vi "svx_Waterfall Facade.vi"(0 "Data In":T3={"z0"=0.0, "dz"=1.0, "Plots"=[]}, 2 "Display State In":T6={"X Scale Width %"=50.0, "Y Scale Height %"=50.0, "X-Axis Range"={"Minimum"=0.0, "Maximum"=10.0}, "Y-Axis Range"={"Minimum"=0.0, "Maximum"=10.0}, "Z-Axis Range"={"Minimum"=0.0, "Maximum"=10.0}, "Plot Color"=61212, "Frame Color"=16252785, "Background Color"=16777222, "Initial AutoScale Y"=TRUE, "AutoScale X"=2, "AutoScale Y"=2, "AutoScale Z"=2, "Plot Transparency"=FALSE, "X-Axis Name"="Frequency", "Y-Axis Name"="Amplitude", "Z-Axis Name"="", "X-Axis Scaling Factor"={"Offset"=0.0, "Multiplier"=1.0}, "Y-Axis Scaling Factor"={"Offset"=0.0, "Multiplier"=1.0}, "Z-Axis Scaling Factor"={"Offset"=0.0, "Multiplier"=1.0}, "X-Scale Visible"=TRUE, "Y-Scale Visible"=TRUE, "Z-Scale Visible"=TRUE, "X-Scale Label Visible"=TRUE, "Y-Scale Label Visible"=TRUE, "Z-Scale Label Visible"=TRUE, "X-Axis Range Scaled"={"Minimum"=0.0, "Maximum"=10.0}, "Y-Axis Range Scaled"={"Minimum"=0.0, "Maximum"=10.0}, "Z-Axis Range Scaled"={"Minimum"=0.0, "Maximum"=10.0}, "Rev Z Order"=FALSE, "X-Scale Format Str"="%#.4g", "Y-Scale Format Str"="%#.4g", "Z-Scale Format Str"="%#.4g", "Decor color"=12369084, "Scale Range Change"=refnum, "out of state queue"=refnum, "property nodes"=refnum, "Lines"=[], "Line Properties"={"Line Color"=61212, "Line Width"=61212, "Line Style"=enum."Dash", "DisplayLines"=FALSE}} {"Line Properties"."Line Width" min=1}, 3 "Container State":T7) -> (6 "Data Out":T3={"z0"=0.0, "dz"=1.0, "Plots"=[]}, 7 "Display State Out":T6={"X Scale Width %"=50.0, "Y Scale Height %"=50.0, "X-Axis Range"={"Minimum"=0.0, "Maximum"=10.0}, "Y-Axis Range"={"Minimum"=0.0, "Maximum"=10.0}, "Z-Axis Range"={"Minimum"=0.0, "Maximum"=10.0}, "Plot Color"=61212, "Frame Color"=16252785, "Background Color"=16777222, "Initial AutoScale Y"=TRUE, "AutoScale X"=2, "AutoScale Y"=2, "AutoScale Z"=2, "Plot Transparency"=FALSE, "X-Axis Name"="Frequency", "Y-Axis Name"="Amplitude", "Z-Axis Name"="", "X-Axis Scaling Factor"={"Offset"=0.0, "Multiplier"=1.0}, "Y-Axis Scaling Factor"={"Offset"=0.0, "Multiplier"=1.0}, "Z-Axis Scaling Factor"={"Offset"=0.0, "Multiplier"=1.0}, "X-Scale Visible"=TRUE, "Y-Scale Visible"=TRUE, "Z-Scale Visible"=TRUE, "X-Scale Label Visible"=TRUE, "Y-Scale Label Visible"=TRUE, "Z-Scale Label Visible"=TRUE, "X-Axis Range Scaled"={"Minimum"=0.0, "Maximum"=10.0}, "Y-Axis Range Scaled"={"Minimum"=0.0, "Maximum"=10.0}, "Z-Axis Range Scaled"={"Minimum"=0.0, "Maximum"=10.0}, "Rev Z Order"=FALSE, "X-Scale Format Str"="%#.4g", "Y-Scale Format Str"="%#.4g", "Z-Scale Format Str"="%#.4g", "Decor color"=12369084, "Scale Range Change"=refnum, "out of state queue"=refnum, "property nodes"=refnum, "Lines"=[], "Line Properties"={"Line Color"=61212, "Line Width"=61212, "Line Style"=enum."Dash", "DisplayLines"=FALSE}} {"Line Properties"."Line Width" min=1}, 8 "Action":T5)   [LabVIEW 2017, in "SVX Waterfall Graph.xctl"]
uses:
  <vilib>/addons/_XControls/Waterfall Graph/SVX Waterfall Graph.xctl
  <vilib>/addons/_XControls/Waterfall Graph/subVIs/svx_Waterfall Data.ctl
  <vilib>/_xctls/Container State.ctl
  <vilib>/addons/_XControls/Waterfall Graph/subVIs/svx_Waterfall State.ctl
  <vilib>/addons/_NISVFA/_Shared subVIs/Controls/svc_Cluster of Array of Cluster of XYZ.ctl
  <vilib>/_xctls/Action.ctl
  <vilib>/addons/_XControls/Waterfall Graph/subVIs/svx_CroppedData.ctl
  <vilib>/Utility/miscctls.llb/LVPoint32TypeDef.ctl
  <vilib>/addons/_XControls/Waterfall Graph/subVIs/svx_Waterfall Execution Tasks.ctl
  <vilib>/addons/_XControls/Waterfall Graph/subVIs/svx_Waterfall Local Variables.ctl
  <vilib>/Utility/cursorutil.llb/Set Cursor (Icon Pict).vi
  <vilib>/_xctls/XControlSupport.lvlib
panel:
  out "Coords":T1
  out "Dec/Cropped and Lines":T2={"Dec/Cropped in"={"z0"=0.0, "dz"=1.0, "Plots"=[]}, "Lines"=[]}
  out "XY Graph":cluster{"X":dbl[], "Y":dbl[]}[](graph)
  out "Z Scale Graph":cluster{"f0":dbl, "df":dbl, "magnitude":dbl[]}[](graph)
  out "XY Scale Graph":cluster{"f0":dbl, "df":dbl, "magnitude":dbl[]}[](graph)
  out "background":bool
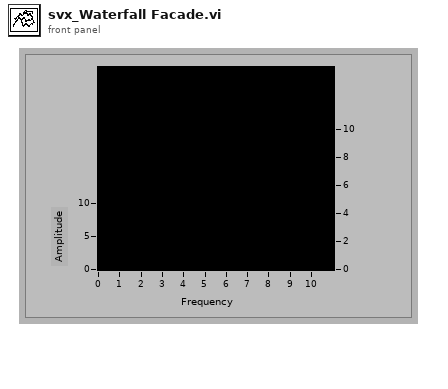
[diagram p1: front panel]
types:
  T1 = typedef "LVPoint32TypeDef.ctl" = cluster{"Horizontal":i32, "Vertical":i32}
  T2 = typedef "SVX Waterfall Graph.xctl/svx_CroppedData.ctl" = cluster{"Dec/Cropped in":T3, "Lines":T4[]}
  T3 = typedef "SVX Waterfall Graph.xctl/svx_Waterfall Data.ctl" = cluster{"z0":dbl, "dz":dbl, "Plots":cluster{"x0":dbl, "dx":dbl, "Y":dbl[]}[]}
  T4 = typedef "svc_Cluster of Array of Cluster of XYZ.ctl" = cluster{"line":cluster{"X":dbl, "Y":dbl, "Z":dbl}[]}
  T5 = typedef "XControlSupport.lvlib/Action.ctl" = cluster{"Data Changed?":bool, "State Changed?":bool, "Action Name":string}
  T6 = typedef "SVX Waterfall Graph.xctl/svx_Waterfall State.ctl" = cluster{"X Scale Width %":dbl, "Y Scale Height %":dbl, "X-Axis Range":cluster{"Minimum":dbl, "Maximum":dbl}, "Y-Axis Range":cluster{"Minimum":dbl, "Maximum":dbl}, "Z-Axis Range":cluster{"Minimum":dbl, "Maximum":dbl}, "Plot Color":u32, "Frame Color":u32, "Background Color":u32, "Initial AutoScale Y":bool, "AutoScale X":u8, "AutoScale Y":u8, "AutoScale Z":u8, "Plot Transparency":bool, "X-Axis Name":string, "Y-Axis Name":string, "Z-Axis Name":string, "X-Axis Scaling Factor":cluster{"Offset":dbl, "Multiplier":dbl}, "Y-Axis Scaling Factor":cluster{"Offset":dbl, "Multiplier":dbl}, "Z-Axis Scaling Factor":cluster{"Offset":dbl, "Multiplier":dbl}, "X-Scale Visible":bool, "Y-Scale Visible":bool, "Z-Scale Visible":bool, "X-Scale Label Visible":bool, "Y-Scale Label Visible":bool, "Z-Scale Label Visible":bool, "X-Axis Range Scaled":cluster{"Minimum":dbl, "Maximum":dbl}, "Y-Axis Range Scaled":cluster{"Minimum":dbl, "Maximum":dbl}, "Z-Axis Range Scaled":cluster{"Minimum":dbl, "Maximum":dbl}, "Rev Z Order":bool, "X-Scale Format Str":string, "Y-Scale Format Str":string, "Z-Scale Format Str":string, "Decor color":u32, "Scale Range Change":refnum<user-event>, "out of state queue":refnum<queue>, "property nodes":refnum<queue>, "Lines":T4[], "Line Properties":cluster{"Line Color":u32, "Line Width":u16, "Line Style":enum32{"Solid", "Dash", "Dot", "DashDot", "DashDotDot"}, "DisplayLines":bool}}
  T7 = typedef "XControlSupport.lvlib/Container State.ctl" = cluster{"Indicator?":bool, "Run Mode?":bool, " Refnum":refnum<vi>}
  T8 = typedef "SVX Waterfall Graph.xctl/svx_Waterfall Local Variables.ctl" = cluster{"Grabbing?":bool, "Coords":T1, "Time":u32}
  T9 = typedef "SVX Waterfall Graph.xctl/svx_Waterfall Execution Tasks.ctl" = enum16{"[Data] Default", "[Data] Update Graph", "[Pane] Calculate Size from Coord Change", "[Pane] Calculate Size from Display State", "[Plot] Redraw Frame", "[Plot] Update Plot Color", "[Scale] Autoscale or Crop X, Y, Z", "[Scale] Resize Scales", "[Scale] Align Scale Labels", "[Plot] Initialize Plot", "[Scale] X Scale", "[Scale] Y Scale", "[Scale] Z Scale", "[Scale] Multiplier/Offset", "[Scale] Name", "[Scale] Visible", "[Scale] Label Visible", "[Scale] Format"}
  T10 = cluster{"use queue?":bool, "X-Axis Range":cluster{"Minimum":dbl, "Maximum":dbl}, "Y-Axis Range":cluster{"Minimum":dbl, "Maximum":dbl}, "Z-Axis Range":cluster{"Minimum":dbl, "Maximum":dbl}, "X-Axis Range Scaled":cluster{"Minimum":dbl, "Maximum":dbl}, "Y-Axis Range Scaled":cluster{"Minimum":dbl, "Maximum":dbl}, "Z-Axis Range Scaled":cluster{"Minimum":dbl, "Maximum":dbl}, "AutoScale X":u8, "AutoScale Y":u8, "AutoScale Z":u8, "background":refnum<vi>}
  T11 = cluster{"Scaled.Minimum":dbl, "Scaled.Maximum":dbl, "Kind":enum16{"X-Scale", "Y-Scale", "Z-Scale"}}
  T12 = cluster{"Range.Minimum":dbl, "Range.Maximum":dbl, "Kind":enum16{"X-Scale", "Y-Scale", "Z-Scale"}}
  T13 = typedef "LVRectTypeDef.ctl" = cluster{"Left":i16, "Top":i16, "Right":i16, "Bottom":i16}
  T14 = typedef "LVPositionTypeDef.ctl" = cluster{"Left":i32, "Top":i32}
  T15 = cluster{"Shift":bool, "Ctrl":bool, "Alt":bool, "Cmd":bool, "Opt":bool}
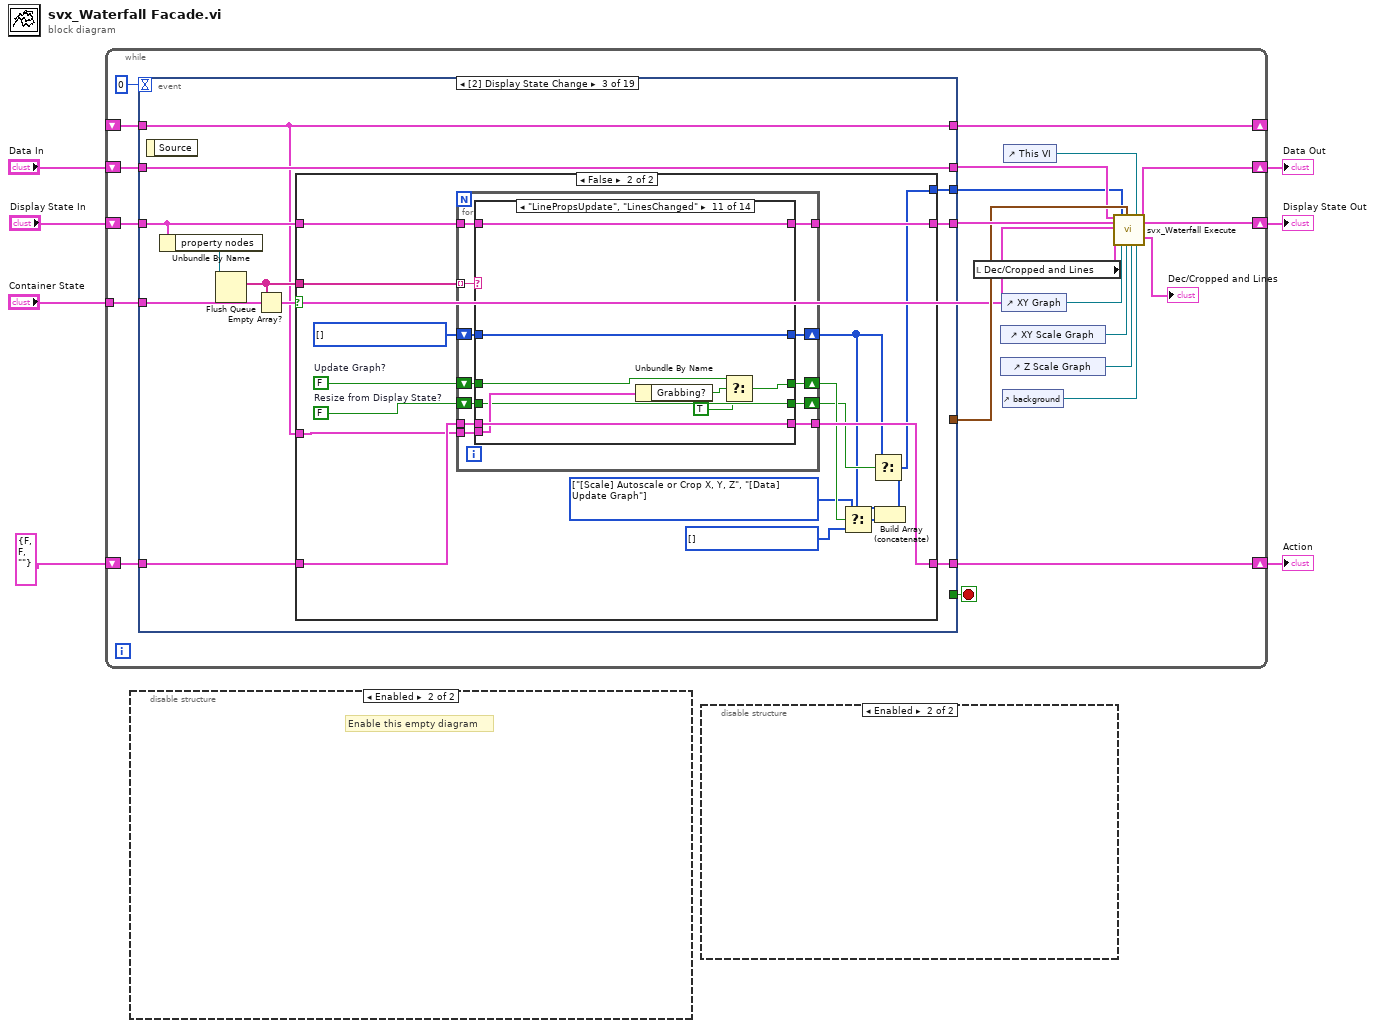
[diagram p0: block diagram]
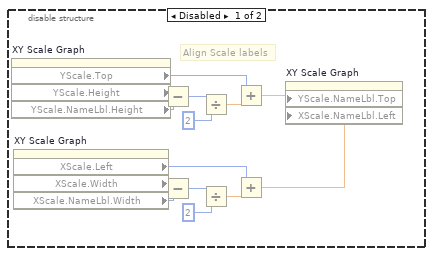
[diagram p2: hidden frame]
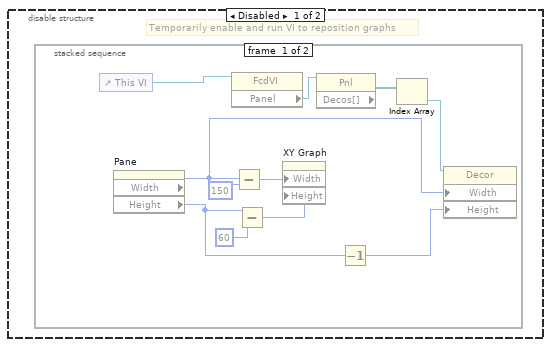
[diagram p3: hidden frame]
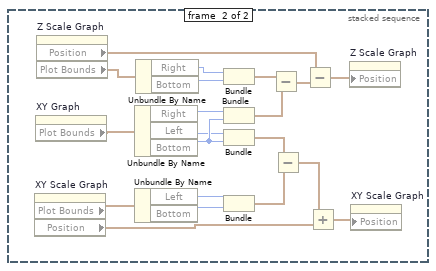
[diagram p4: hidden frame]
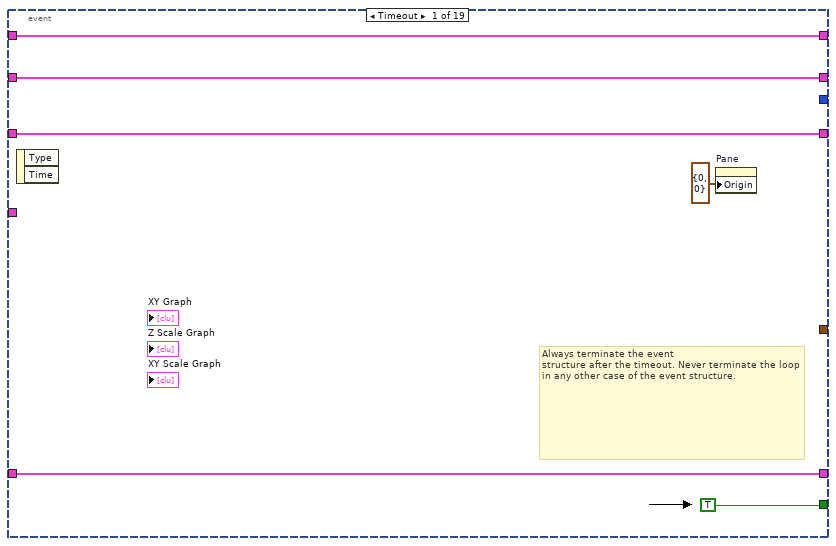
[diagram p5: hidden frame]
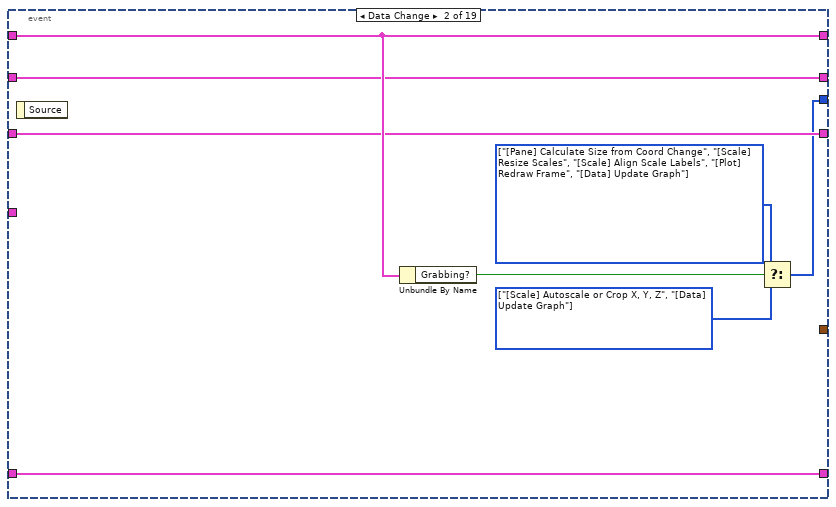
[diagram p6: hidden frame]
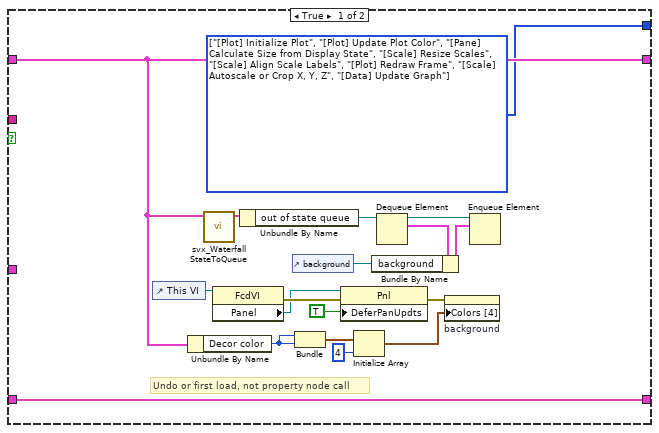
[diagram p7: hidden frame]
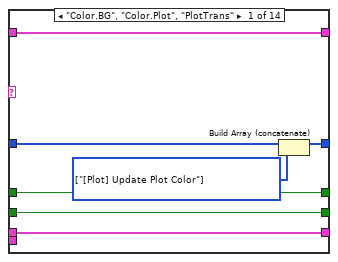
[diagram p8: hidden frame]
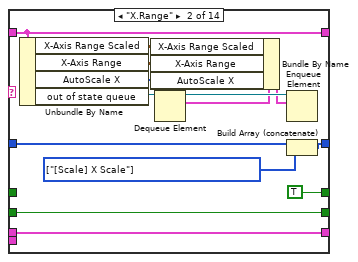
[diagram p9: hidden frame]
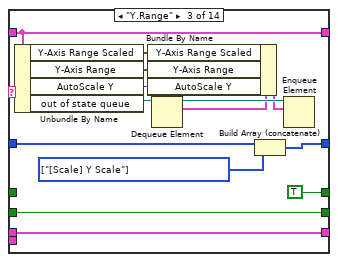
[diagram p10: hidden frame]
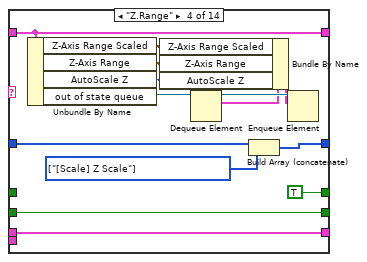
[diagram p11: hidden frame]
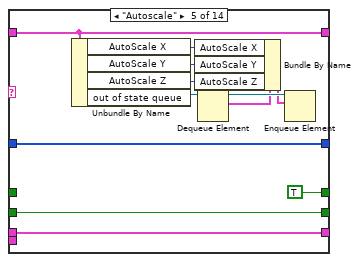
[diagram p12: hidden frame]
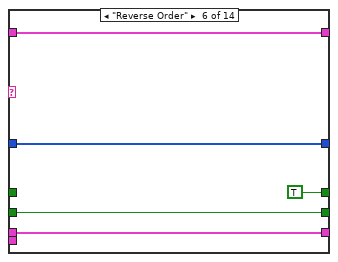
[diagram p13: hidden frame]
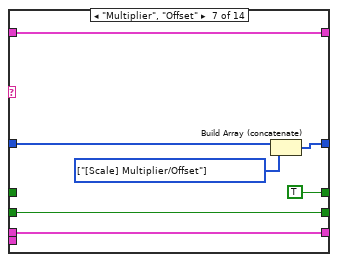
[diagram p14: hidden frame]
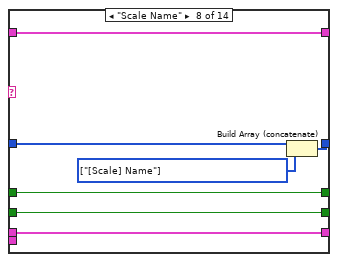
[diagram p15: hidden frame]
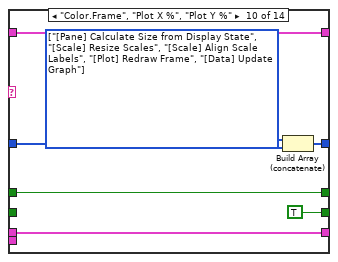
[diagram p17: hidden frame]
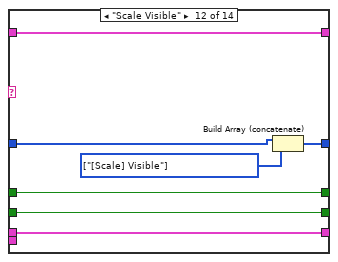
[diagram p18: hidden frame]
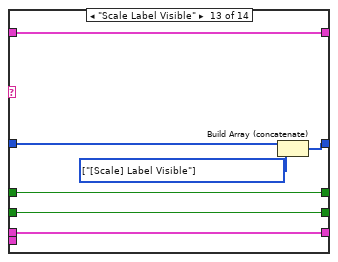
[diagram p19: hidden frame]
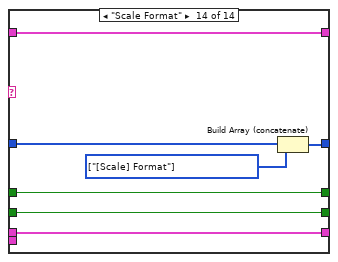
[diagram p20: hidden frame]
diagram:
  n1 = while {
    shift-right: [w18] -> w4
    shift-left: "Display State In" -> [w29]
    tunnel: "Container State" -> [w21]
    shift-right: [w10] -> w7
    shift-left: "Data In" -> [w26]
    shift-right: [w9] -> w2
    shift-left: T5 {"Data Changed?"=FALSE, "State Changed?"=FALSE, "Action Name"=""} ("Action") -> [w25]
    shift-right: [w19] -> _
    shift-left: _ -> [w24]
    stop <- w28 stop-if-true
    n2 = event shown="[2] Display State Change" {
      selector: _ -> [_ _ _ _ _ _ _ _ _ _ _ _ _ _ _ _ _ _ _]
      dyn-events: _ -> [_ _ _ _ _ _ _ _ _ _ _ _ _ _ _ _ _ _ _]
      timeout: 0 -> [_ _ _ _ _ _ _ _ _ _ _ _ _ _ _ _ _ _ _]
      tunnel: w29 -> [w30 w41 w47 w226 w229 w236 w262 w290 w325 w343 w354 w358 w415 w431 w474 w487 w506 w658 w678]
      tunnel: [w30 w41 w53 w226 w229 w235 w262 w290 w325 w343 w353 w358 w415 w431 w474 w487 w505 w658 w678] -> w23
      tunnel: [TRUE _ _ _ _ _ _ _ _ _ _ _ _ _ _ _ _ _ _] -> w28
      tunnel: w21 -> [_ _ _ w227 w232 w241 _ w289 w320 _ _ _ _ _ w473 w483 w501 _ _]
      tunnel: w26 -> [w34 w42 w45 w225 w231 w237 w265 w294 w324 w344 w355 w371 w425 w433 w480 w490 w502 w655 w679]
      tunnel: [w34 w42 w45 w225 w231 w237 w265 w294 w324 w344 w355 w371 w425 w433 w480 w490 w502 w654 w679] -> w20
      tunnel: [w31 w40 w52 w224 w228 w238 w261 w287 w318 w342 w351 w373 w426 w432 w481 w491 w503 w652 w677] -> w9
      tunnel: w25 -> [w31 w40 w51 w224 w228 w239 w261 w288 w319 w342 w352 w374 w427 w432 w481 w491 w504 w653 w677]
      tunnel: [w32 w43 w44 w223 w230 w249 w275 w297 w323 w345 w356 w376 w429 w435 w479 w489 w507 w659 w680] -> w19
      tunnel: w24 -> [w32 w43 w44 w223 w230 _ w274 w296 w322 w345 w356 w376 w429 w435 w479 w489 w507 w659 w680]
      tunnel: [_ _ _ _ _ _ w263 w291 _ _ _ _ _ _ _ _ _ _ _] -> w22
      tunnel: [_ w36 w46 _ _ _ w260 w286 w317 _ _ w357 w414 w430 _ _ w500 w651 _] -> w17
      event Timeout {
        # "Always terminate the event\nstructure after the timeout. Never terminate the loop in any other case of the event structure."
        n3 = event-data() -> ()  [unwired: 1 in, 2 out]
        n4 = property on="Pane" class="Pane"("Origin"=cluster{"Horizontal":i16, "Vertical":i16} {"Horizontal"=0, "Vertical"=0}) -> ()  [unwired: 2 in, 2 out]
      }
      event Data Change {
        w38 = T9[] [enum."[Scale] Autoscale or Crop X, Y, Z", enum."[Data] Update Graph"] items=["[Data] Default", "[Data] Update Graph", "[Pane] Calculate Size from Coord Change", "[Pane] Calculate Size from Display State", "[Plot] Redraw Frame", "[Plot] Update Plot Color", "[Scale] Autoscale or Crop X, Y, Z", "[Scale] Resize Scales", "[Scale] Align Scale Labels", "[Plot] Initialize Plot", "[Scale] X Scale", "[Scale] Y Scale", "[Scale] Z Scale", "[Scale] Multiplier/Offset", "[Scale] Name", "[Scale] Visible", "[Scale] Label Visible", "[Scale] Format"] ("Execution Tasks")
        w39 = T9[] [enum."[Pane] Calculate Size from Coord Change", enum."[Scale] Resize Scales", enum."[Scale] Align Scale Labels", enum."[Plot] Redraw Frame", enum."[Data] Update Graph"] items=["[Data] Default", "[Data] Update Graph", "[Pane] Calculate Size from Coord Change", "[Pane] Calculate Size from Display State", "[Plot] Redraw Frame", "[Plot] Update Plot Color", "[Scale] Autoscale or Crop X, Y, Z", "[Scale] Resize Scales", "[Scale] Align Scale Labels", "[Plot] Initialize Plot", "[Scale] X Scale", "[Scale] Y Scale", "[Scale] Z Scale", "[Scale] Multiplier/Offset", "[Scale] Name", "[Scale] Visible", "[Scale] Label Visible", "[Scale] Format"] ("Execution Tasks")
        n5 = event-data() -> ()  [unwired: 1 in, 1 out]
        n6 = Unbundle By Name(w43) -> ("Grabbing?"=w37:bool)
        n7 = Select(t=w39, s=w37, f=w38) -> (s? t:f=w36:T9[])
      }
      event Display State Change {
        n8 = event-data() -> ()  [unwired: 1 in, 1 out]
        n9 = Unbundle By Name(w47) -> ("property nodes"=w49:refnum<queue>)
        n10 = Flush Queue(queue=w49) -> (remaining elements=w48:string[])  [unwired: 1 in, 2 out]
        n11 = Empty Array?(array=w48) -> (empty?=w50:bool)
        n12 = case shown="False" w50 {
          tunnel: [w71 w88] -> w53
          tunnel: [w55 w87] -> w52
          tunnel: w47 -> [w71 w86]
          tunnel: w51 -> [w55 w85]
          tunnel: w48 -> [_ w84]
          tunnel: [w54 w76] -> w46
          tunnel: w44 -> [_ w72]
          frame True {
            w54 = T9[] [enum."[Plot] Initialize Plot", enum."[Plot] Update Plot Color", enum."[Pane] Calculate Size from Display State", enum."[Scale] Resize Scales", enum."[Scale] Align Scale Labels", enum."[Plot] Redraw Frame", enum."[Scale] Autoscale or Crop X, Y, Z", enum."[Data] Update Graph"] items=["[Data] Default", "[Data] Update Graph", "[Pane] Calculate Size from Coord Change", "[Pane] Calculate Size from Display State", "[Plot] Redraw Frame", "[Plot] Update Plot Color", "[Scale] Autoscale or Crop X, Y, Z", "[Scale] Resize Scales", "[Scale] Align Scale Labels", "[Plot] Initialize Plot", "[Scale] X Scale", "[Scale] Y Scale", "[Scale] Z Scale", "[Scale] Multiplier/Offset", "[Scale] Name", "[Scale] Visible", "[Scale] Label Visible", "[Scale] Format"] ("Execution Tasks")
            # "Undo or first load, not property node call"
            n13 = control-ref of="This VI"() -> (w57:refnum<vi>)
            n14 = Unbundle By Name(w71) -> ("Decor color"=w70:u32)
            n15 = call <vilib>:"svx_Waterfall StateToQueue.vi"("Display State In"=w71) -> ("Display State Out"=w66:T6)  [unwired: 10 in]
            n16 = property class="FcdVI"(reference=w57) -> (error out=w60:errorcluster, "Panel"=w58:refnum<vi>)  [unwired: 1 in, 1 out]
            n17 = Unbundle By Name(w66) -> ("out of state queue"=w65:refnum<queue>)
            n18 = control-ref of="background"() -> (w61:refnum<vi>)
            n19 = Bundle("Decor color"=w70, "Decor color"=w70) -> (w69:cluster{"Decor color":u32, "Decor color":u32})  [unwired: 1 in]
            n20 = property class="Pnl"(reference=w58, error in=w60, "DeferPanUpdts"=TRUE ("Defer Panel Updates")) -> (error out=w56:errorcluster)  [unwired: 1 out]
            n21 = Initialize Array(w69, 4 ("dimension size")) -> (w67:cluster{"Decor color":u32, "Decor color":u32}[])
            n22 = Dequeue Element(queue=w65) -> (queue out=w64:refnum<queue>, element=w63:T10)  [unwired: 2 in, 2 out]
            n23 = Bundle By Name(cluster=w63, "background"=w61) -> (w62:T10)
            n24 = property on="background" class="Bool"(error in=w56, "Colors [4]"=w67) -> ()  [unwired: 1 in, 2 out]
            n25 = Enqueue Element(queue=w64, element=w62) -> ()  [unwired: 2 in, 3 out]
          }
          frame False {
            w78 = T9[] [] items=["[Data] Default", "[Data] Update Graph", "[Pane] Calculate Size from Coord Change", "[Pane] Calculate Size from Display State", "[Plot] Redraw Frame", "[Plot] Update Plot Color", "[Scale] Autoscale or Crop X, Y, Z", "[Scale] Resize Scales", "[Scale] Align Scale Labels", "[Plot] Initialize Plot", "[Scale] X Scale", "[Scale] Y Scale", "[Scale] Z Scale", "[Scale] Multiplier/Offset", "[Scale] Name", "[Scale] Visible", "[Scale] Label Visible", "[Scale] Format"] ("Execution Tasks")
            w79 = T9[] [enum."[Scale] Autoscale or Crop X, Y, Z", enum."[Data] Update Graph"] items=["[Data] Default", "[Data] Update Graph", "[Pane] Calculate Size from Coord Change", "[Pane] Calculate Size from Display State", "[Plot] Redraw Frame", "[Plot] Update Plot Color", "[Scale] Autoscale or Crop X, Y, Z", "[Scale] Resize Scales", "[Scale] Align Scale Labels", "[Plot] Initialize Plot", "[Scale] X Scale", "[Scale] Y Scale", "[Scale] Z Scale", "[Scale] Multiplier/Offset", "[Scale] Name", "[Scale] Visible", "[Scale] Label Visible", "[Scale] Format"] ("Execution Tasks")
            w83 = T9[] [] items=["[Data] Default", "[Data] Update Graph", "[Pane] Calculate Size from Coord Change", "[Pane] Calculate Size from Display State", "[Plot] Redraw Frame", "[Plot] Update Plot Color", "[Scale] Autoscale or Crop X, Y, Z", "[Scale] Resize Scales", "[Scale] Align Scale Labels", "[Plot] Initialize Plot", "[Scale] X Scale", "[Scale] Y Scale", "[Scale] Z Scale", "[Scale] Multiplier/Offset", "[Scale] Name", "[Scale] Visible", "[Scale] Label Visible", "[Scale] Format"] ("Execution Tasks")
            w81 = FALSE  # Resize from Display State?
            w82 = FALSE  # Update Graph?
            n26 = for {
              tunnel: [w100] -> w88
              tunnel: [w99] -> w87
              tunnel: w86 -> [w98]
              tunnel: w85 -> [w97]
              tunnel: w84 -> [w96] mode=indexing
              shift-right: [w94] -> w74
              shift-left: w83 -> [w95]
              shift-right: [w92] -> w80
              shift-left: w82 -> [w93]
              shift-right: [w90] -> w77
              shift-left: w81 -> [w91]
              tunnel: w72 -> [w89]
              n27 = case shown="\"LinePropsUpdate\", \"LinesChanged\"" w96 {
                tunnel: [w106 w120 w134 w148 w158 w165 w172 w179 w185 w191 w201 w207 w214 w221] -> w100
                tunnel: [w107 w121 w135 w149 w161 w166 w173 w180 w184 w192 w200 w208 w215 w222] -> w99
                tunnel: w98 -> [w106 w120 w134 w148 w158 w165 w172 w179 w185 w191 w201 w207 w214 w221]
                tunnel: w97 -> [w107 w121 w135 w149 w161 w166 w173 w180 w184 w192 w200 w208 w215 w222]
                tunnel: w95 -> [w105 w110 w125 w139 w152 w164 w169 w177 w183 w189 w197 w203 w211 w217]
                tunnel: [w104 w109 w124 w138 w152 w164 w170 w176 w183 w188 w197 w204 w210 w218] -> w94
                tunnel: w93 -> [w102 _ _ _ _ _ _ w175 w182 w187 w195 w206 w213 w220]
                tunnel: [w102 TRUE ("Update Graph?") TRUE ("Update Graph?") TRUE ("Update Graph?") TRUE ("Update Graph?") TRUE ("Update Graph?") TRUE ("Update Graph?") w175 w182 w187 w194 w206 w213 w220] -> w92
                tunnel: w91 -> [w101 w108 w122 w136 w150 w162 w167 w174 w181 _ w198 w202 w209 w216]
                tunnel: [w101 w108 w122 w136 w150 w162 w167 w174 w181 TRUE ("Resize from Display State?") w198 w202 w209 w216] -> w90
                tunnel: w89 -> [_ _ _ _ _ _ _ _ _ _ w199 _ _ _]
                frame "Color.BG", "Color.Plot", "PlotTrans" {
                  w103 = T9[] [enum."[Plot] Update Plot Color"] items=["[Data] Default", "[Data] Update Graph", "[Pane] Calculate Size from Coord Change", "[Pane] Calculate Size from Display State", "[Plot] Redraw Frame", "[Plot] Update Plot Color", "[Scale] Autoscale or Crop X, Y, Z", "[Scale] Resize Scales", "[Scale] Align Scale Labels", "[Plot] Initialize Plot", "[Scale] X Scale", "[Scale] Y Scale", "[Scale] Z Scale", "[Scale] Multiplier/Offset", "[Scale] Name", "[Scale] Visible", "[Scale] Label Visible", "[Scale] Format"] ("Execution Tasks")
                  n28 = Build Array (concatenate)(w105, w103) -> (w104:T9[])
                }
                frame "X.Range" {
                  w111 = T9[] [enum."[Scale] X Scale"] items=["[Data] Default", "[Data] Update Graph", "[Pane] Calculate Size from Coord Change", "[Pane] Calculate Size from Display State", "[Plot] Redraw Frame", "[Plot] Update Plot Color", "[Scale] Autoscale or Crop X, Y, Z", "[Scale] Resize Scales", "[Scale] Align Scale Labels", "[Plot] Initialize Plot", "[Scale] X Scale", "[Scale] Y Scale", "[Scale] Z Scale", "[Scale] Multiplier/Offset", "[Scale] Name", "[Scale] Visible", "[Scale] Label Visible", "[Scale] Format"] ("Execution Tasks")
                  n29 = Unbundle By Name(w120) -> ("X-Axis Range Scaled"=w115:cluster{"Minimum":dbl, "Maximum":dbl}, "X-Axis Range"=w113:cluster{"Minimum":dbl, "Maximum":dbl}, "AutoScale X"=w114:u8, "out of state queue"=w119:refnum<queue>)
                  n30 = Dequeue Element(queue=w119) -> (queue out=w118:refnum<queue>, element=w117:T10)  [unwired: 2 in, 2 out]
                  n31 = Bundle By Name(cluster=w117, "X-Axis Range Scaled"=w115, "X-Axis Range"=w113, "AutoScale X"=w114) -> (w116:T10)
                  n32 = Enqueue Element(queue=w118, element=w116) -> ()  [unwired: 2 in, 3 out]
                  n33 = Build Array (concatenate)(w110, w111) -> (w109:T9[])
                }
                frame "Y.Range" {
                  w126 = T9[] [enum."[Scale] Y Scale"] items=["[Data] Default", "[Data] Update Graph", "[Pane] Calculate Size from Coord Change", "[Pane] Calculate Size from Display State", "[Plot] Redraw Frame", "[Plot] Update Plot Color", "[Scale] Autoscale or Crop X, Y, Z", "[Scale] Resize Scales", "[Scale] Align Scale Labels", "[Plot] Initialize Plot", "[Scale] X Scale", "[Scale] Y Scale", "[Scale] Z Scale", "[Scale] Multiplier/Offset", "[Scale] Name", "[Scale] Visible", "[Scale] Label Visible", "[Scale] Format"] ("Execution Tasks")
                  n34 = Unbundle By Name(w134) -> ("Y-Axis Range Scaled"=w133:cluster{"Minimum":dbl, "Maximum":dbl}, "Y-Axis Range"=w128:cluster{"Minimum":dbl, "Maximum":dbl}, "AutoScale Y"=w127:u8, "out of state queue"=w131:refnum<queue>)
                  n35 = Dequeue Element(queue=w131) -> (queue out=w132:refnum<queue>, element=w130:T10)  [unwired: 2 in, 2 out]
                  n36 = Bundle By Name(cluster=w130, "Y-Axis Range Scaled"=w133, "Y-Axis Range"=w128, "AutoScale Y"=w127) -> (w129:T10)
                  n37 = Build Array (concatenate)(w125, w126) -> (w124:T9[])
                  n38 = Enqueue Element(queue=w132, element=w129) -> ()  [unwired: 2 in, 3 out]
                }
                frame "Z.Range" {
                  w140 = T9[] [enum."[Scale] Z Scale"] items=["[Data] Default", "[Data] Update Graph", "[Pane] Calculate Size from Coord Change", "[Pane] Calculate Size from Display State", "[Plot] Redraw Frame", "[Plot] Update Plot Color", "[Scale] Autoscale or Crop X, Y, Z", "[Scale] Resize Scales", "[Scale] Align Scale Labels", "[Plot] Initialize Plot", "[Scale] X Scale", "[Scale] Y Scale", "[Scale] Z Scale", "[Scale] Multiplier/Offset", "[Scale] Name", "[Scale] Visible", "[Scale] Label Visible", "[Scale] Format"] ("Execution Tasks")
                  n39 = Unbundle By Name(w148) -> ("Z-Axis Range Scaled"=w144:cluster{"Minimum":dbl, "Maximum":dbl}, "Z-Axis Range"=w143:cluster{"Minimum":dbl, "Maximum":dbl}, "AutoScale Z"=w145:u8, "out of state queue"=w146:refnum<queue>)
                  n40 = Dequeue Element(queue=w146) -> (queue out=w147:refnum<queue>, element=w142:T10)  [unwired: 2 in, 2 out]
                  n41 = Bundle By Name(cluster=w142, "Z-Axis Range Scaled"=w144, "Z-Axis Range"=w143, "AutoScale Z"=w145) -> (w141:T10)
                  n42 = Build Array (concatenate)(w139, w140) -> (w138:T9[])
                  n43 = Enqueue Element(queue=w147, element=w141) -> ()  [unwired: 2 in, 3 out]
                }
                frame "Autoscale" {
                  n44 = Unbundle By Name(w158) -> ("AutoScale X"=w155:u8, "AutoScale Y"=w154:u8, "AutoScale Z"=w153:u8, "out of state queue"=w159:refnum<queue>)
                  n45 = Dequeue Element(queue=w159) -> (queue out=w160:refnum<queue>, element=w157:T10)  [unwired: 2 in, 2 out]
                  n46 = Bundle By Name(cluster=w157, "AutoScale X"=w155, "AutoScale Y"=w154, "AutoScale Z"=w153) -> (w156:T10)
                  n47 = Enqueue Element(queue=w160, element=w156) -> ()  [unwired: 2 in, 3 out]
                }
                frame "Reverse Order" {
                }
                frame "Multiplier", "Offset" {
                  w171 = T9[] [enum."[Scale] Multiplier/Offset"] items=["[Data] Default", "[Data] Update Graph", "[Pane] Calculate Size from Coord Change", "[Pane] Calculate Size from Display State", "[Plot] Redraw Frame", "[Plot] Update Plot Color", "[Scale] Autoscale or Crop X, Y, Z", "[Scale] Resize Scales", "[Scale] Align Scale Labels", "[Plot] Initialize Plot", "[Scale] X Scale", "[Scale] Y Scale", "[Scale] Z Scale", "[Scale] Multiplier/Offset", "[Scale] Name", "[Scale] Visible", "[Scale] Label Visible", "[Scale] Format"] ("Execution Tasks")
                  n48 = Build Array (concatenate)(w169, w171) -> (w170:T9[])
                }
                frame "Scale Name" {
                  w178 = T9[] [enum."[Scale] Name"] items=["[Data] Default", "[Data] Update Graph", "[Pane] Calculate Size from Coord Change", "[Pane] Calculate Size from Display State", "[Plot] Redraw Frame", "[Plot] Update Plot Color", "[Scale] Autoscale or Crop X, Y, Z", "[Scale] Resize Scales", "[Scale] Align Scale Labels", "[Plot] Initialize Plot", "[Scale] X Scale", "[Scale] Y Scale", "[Scale] Z Scale", "[Scale] Multiplier/Offset", "[Scale] Name", "[Scale] Visible", "[Scale] Label Visible", "[Scale] Format"] ("Execution Tasks")
                  n49 = Build Array (concatenate)(w177, w178) -> (w176:T9[])
                }
                frame Default {
                }
                frame "Color.Frame", "Plot X %", "Plot Y %" {
                  w190 = T9[] [enum."[Pane] Calculate Size from Display State", enum."[Scale] Resize Scales", enum."[Scale] Align Scale Labels", enum."[Plot] Redraw Frame", enum."[Data] Update Graph"] items=["[Data] Default", "[Data] Update Graph", "[Pane] Calculate Size from Coord Change", "[Pane] Calculate Size from Display State", "[Plot] Redraw Frame", "[Plot] Update Plot Color", "[Scale] Autoscale or Crop X, Y, Z", "[Scale] Resize Scales", "[Scale] Align Scale Labels", "[Plot] Initialize Plot", "[Scale] X Scale", "[Scale] Y Scale", "[Scale] Z Scale", "[Scale] Multiplier/Offset", "[Scale] Name", "[Scale] Visible", "[Scale] Label Visible", "[Scale] Format"] ("Execution Tasks")
                  n50 = Build Array (concatenate)(w189, w190) -> (w188:T9[])
                }
                frame "LinePropsUpdate", "LinesChanged" {
                  n51 = Unbundle By Name(w199) -> ("Grabbing?"=w196:bool)
                  n52 = Select(t=w195, s=w196, f=TRUE) -> (s? t:f=w194:bool)
                }
                frame "Scale Visible" {
                  w205 = T9[] [enum."[Scale] Visible"] items=["[Data] Default", "[Data] Update Graph", "[Pane] Calculate Size from Coord Change", "[Pane] Calculate Size from Display State", "[Plot] Redraw Frame", "[Plot] Update Plot Color", "[Scale] Autoscale or Crop X, Y, Z", "[Scale] Resize Scales", "[Scale] Align Scale Labels", "[Plot] Initialize Plot", "[Scale] X Scale", "[Scale] Y Scale", "[Scale] Z Scale", "[Scale] Multiplier/Offset", "[Scale] Name", "[Scale] Visible", "[Scale] Label Visible", "[Scale] Format"] ("Execution Tasks")
                  n53 = Build Array (concatenate)(w203, w205) -> (w204:T9[])
                }
                frame "Scale Label Visible" {
                  w212 = T9[] [enum."[Scale] Label Visible"] items=["[Data] Default", "[Data] Update Graph", "[Pane] Calculate Size from Coord Change", "[Pane] Calculate Size from Display State", "[Plot] Redraw Frame", "[Plot] Update Plot Color", "[Scale] Autoscale or Crop X, Y, Z", "[Scale] Resize Scales", "[Scale] Align Scale Labels", "[Plot] Initialize Plot", "[Scale] X Scale", "[Scale] Y Scale", "[Scale] Z Scale", "[Scale] Multiplier/Offset", "[Scale] Name", "[Scale] Visible", "[Scale] Label Visible", "[Scale] Format"] ("Execution Tasks")
                  n54 = Build Array (concatenate)(w211, w212) -> (w210:T9[])
                }
                frame "Scale Format" {
                  w219 = T9[] [enum."[Scale] Format"] items=["[Data] Default", "[Data] Update Graph", "[Pane] Calculate Size from Coord Change", "[Pane] Calculate Size from Display State", "[Plot] Redraw Frame", "[Plot] Update Plot Color", "[Scale] Autoscale or Crop X, Y, Z", "[Scale] Resize Scales", "[Scale] Align Scale Labels", "[Plot] Initialize Plot", "[Scale] X Scale", "[Scale] Y Scale", "[Scale] Z Scale", "[Scale] Multiplier/Offset", "[Scale] Name", "[Scale] Visible", "[Scale] Label Visible", "[Scale] Format"] ("Execution Tasks")
                  n55 = Build Array (concatenate)(w217, w219) -> (w218:T9[])
                }
              }
            }
            n56 = Select(t=w79, s=w80, f=w78) -> (s? t:f=w75:T9[])
            n57 = Build Array (concatenate)(w74, w75) -> (w73:T9[])
            n58 = Select(t=w74, s=w77, f=w73) -> (s? t:f=w76:T9[])
          }
        }
      }
      event Direction Change {
        # "The direction of the XControl changed from a control to an indicator or vice versa. Update the appearance accordingly."
        n59 = event-data() -> ()  [unwired: 1 in, 4 out]
        n60 = Unbundle By Name(w227) -> ()  [unwired: 1 out]
      }
      event Exec State Change {
        # "Handle Edit Mode & Run Mode\ncase differently"
        n61 = event-data() -> ()  [unwired: 1 in, 4 out]
        n62 = Unbundle By Name(w232) -> ()  [unwired: 1 out]
      }
      event "XY Graph": Mouse Down? {
        n63 = event-data() -> ("Coords"=w248:T1, "PlatMods.Ctrl"=w244:bool, "Button"=w246:u16)  [unwired: 1 in]
        n64 = Equal?(x=w246, y=u16 1) -> (x = y?=w243:bool)
        n65 = And(x=w244, y=w243) -> (x .and. y?=w242:bool)
        n66 = case shown="True" w242 {
          tunnel: [w250 w259] -> w249
          tunnel: w248 -> [_ w257]
          tunnel: T8 {"Grabbing?"=FALSE, "Coords"={"Horizontal"=0, "Vertical"=0}, "Time"=0} -> [w250 w256]
          tunnel: w241 -> [_ w255]
          frame False {
          }
          frame True {
            n67 = Unbundle By Name(w255) -> ("Refnum"=w254:refnum<vi>)
            n68 = property class="Ctl"(reference=w254) -> ("OwningVI"=w253:refnum<vi>)  [unwired: 1 in, 2 out]
            n69 = Bundle By Name(cluster=w256, "Grabbing?"=TRUE, "Coords"=w257, "Time"=u32 0) -> (w259:T8)
            n70 = call-poly <vilib>:"Set Cursor.vi"("VI reference (current VI)"=w253, "icon"=u16 11) -> ()  [unwired: 8 in, 2 out]
          }
        }
        n71 = Unbundle By Name(w236) -> ("Background Color"=w240:u32)
        n72 = property on="XY Graph" class="XYGraph (strict)"() -> ("BG Color"=w234:u32)  [unwired: 2 in, 2 out]
        n73 = Not Equal?(x=w234, y=w240) -> (x != y?=w233:bool)
        n74 = Bundle By Name(cluster=w239, "State Changed?"=w233) -> (w238:T5)
        n75 = Bundle By Name(cluster=w236, "Background Color"=w234) -> (w235:T6)
        n76 = event-data() -> ()  [unwired: 2 in, 1 out]
      }
      event "XY Graph": Mouse Move {
        # "Time delay so \nwe don't execute\nevery event"
        n77 = event-data() -> ("Time"=w266:u32, "Coords"=w267:T1)  [unwired: 1 in]
        n78 = Unbundle By Name(w274) -> ("Coords"=w268:T1, "Grabbing?"=w271:bool, "Time"=w273:u32)
        n79 = Subtract(x=w266, y=w273) -> (x-y=w272:u32)
        n80 = Greater Or Equal?(x=w272, y=u32 50 ("delay")) -> (x >= y?=w270:bool)
        n81 = And(x=w271, y=w270) -> (x .and. y?=w269:bool)
        n82 = case shown="True" w269 {
          tunnel: [w278 w285] -> w275
          tunnel: w274 -> [w278 w284]
          tunnel: w268 -> [_ w283]
          tunnel: w267 -> [_ w281]
          tunnel: w266 -> [_ w282]
          tunnel: [cluster{"Horizontal":i32, "Vertical":i32} {"Horizontal"=0, "Vertical"=0} w280] -> w263
          tunnel: [w276 w279] -> w260
          frame False {
            w276 = T9[] [] items=["[Data] Default", "[Data] Update Graph", "[Pane] Calculate Size from Coord Change", "[Pane] Calculate Size from Display State", "[Plot] Redraw Frame", "[Plot] Update Plot Color", "[Scale] Autoscale or Crop X, Y, Z", "[Scale] Resize Scales", "[Scale] Align Scale Labels", "[Plot] Initialize Plot", "[Scale] X Scale", "[Scale] Y Scale", "[Scale] Z Scale", "[Scale] Multiplier/Offset", "[Scale] Name", "[Scale] Visible", "[Scale] Label Visible", "[Scale] Format"] ("Execution Tasks")
          }
          frame True {
            w279 = T9[] [enum."[Pane] Calculate Size from Coord Change", enum."[Scale] Resize Scales", enum."[Scale] Align Scale Labels", enum."[Plot] Redraw Frame", enum."[Data] Update Graph"] items=["[Data] Default", "[Data] Update Graph", "[Pane] Calculate Size from Coord Change", "[Pane] Calculate Size from Display State", "[Plot] Redraw Frame", "[Plot] Update Plot Color", "[Scale] Autoscale or Crop X, Y, Z", "[Scale] Resize Scales", "[Scale] Align Scale Labels", "[Plot] Initialize Plot", "[Scale] X Scale", "[Scale] Y Scale", "[Scale] Z Scale", "[Scale] Multiplier/Offset", "[Scale] Name", "[Scale] Visible", "[Scale] Label Visible", "[Scale] Format"] ("Execution Tasks")
            n83 = Subtract(x=w281, y=w283) -> (x-y=w280:T1)
            n84 = Bundle By Name(cluster=w284, "Time"=w282, "Coords"=w281) -> (w285:T8)
          }
        }
      }
      event "XY Graph": Mouse Up {
        n85 = event-data() -> ("Coords"=w293:T1)  [unwired: 1 in]
        n86 = Unbundle By Name(w296) -> ("Grabbing?"=w295:bool, "Coords"=w292:T1)
        n87 = case shown="True" w295 {
          tunnel: [w301 w313] -> w297
          tunnel: w296 -> [w301 w314]
          tunnel: w293 -> [_ w316]
          tunnel: w292 -> [_ w315]
          tunnel: [cluster{"Horizontal":i32, "Vertical":i32} {"Horizontal"=0, "Vertical"=0} w311] -> w291
          tunnel: w289 -> [_ w307]
          tunnel: w288 -> [w299 w306]
          tunnel: [w299 w305] -> w287
          tunnel: [w298 w302] -> w286
          frame False {
            w298 = T9[] [] items=["[Data] Default", "[Data] Update Graph", "[Pane] Calculate Size from Coord Change", "[Pane] Calculate Size from Display State", "[Plot] Redraw Frame", "[Plot] Update Plot Color", "[Scale] Autoscale or Crop X, Y, Z", "[Scale] Resize Scales", "[Scale] Align Scale Labels", "[Plot] Initialize Plot", "[Scale] X Scale", "[Scale] Y Scale", "[Scale] Z Scale", "[Scale] Multiplier/Offset", "[Scale] Name", "[Scale] Visible", "[Scale] Label Visible", "[Scale] Format"] ("Execution Tasks")
          }
          frame True {
            w302 = T9[] [enum."[Pane] Calculate Size from Coord Change", enum."[Scale] Resize Scales", enum."[Scale] Align Scale Labels", enum."[Plot] Redraw Frame", enum."[Data] Update Graph"] items=["[Data] Default", "[Data] Update Graph", "[Pane] Calculate Size from Coord Change", "[Pane] Calculate Size from Display State", "[Plot] Redraw Frame", "[Plot] Update Plot Color", "[Scale] Autoscale or Crop X, Y, Z", "[Scale] Resize Scales", "[Scale] Align Scale Labels", "[Plot] Initialize Plot", "[Scale] X Scale", "[Scale] Y Scale", "[Scale] Z Scale", "[Scale] Multiplier/Offset", "[Scale] Name", "[Scale] Visible", "[Scale] Label Visible", "[Scale] Format"] ("Execution Tasks")
            n88 = Unbundle By Name(w307) -> ("Refnum"=w310:refnum<vi>)
            n89 = Subtract(x=w316, y=w315) -> (x-y=w311:T1)
            n90 = property class="Ctl"(reference=w310) -> ("OwningVI"=w309:refnum<vi>)  [unwired: 1 in, 2 out]
            n91 = call-poly <vilib>:"Set Cursor.vi"("VI reference (current VI)"=w309, "icon"=u16 0) -> ()  [unwired: 8 in, 2 out]
            n92 = Bundle By Name(cluster=w306, "Action Name"="Perspective Change", "State Changed?"=TRUE) -> (w305:T5)
            n93 = Bundle By Name(cluster=w314, "Grabbing?"=FALSE) -> (w313:T8)
          }
        }
      }
      event "XY Graph": Mouse Leave {
        n94 = event-data() -> ()  [unwired: 1 in, 1 out]
        n95 = Unbundle By Name(w322) -> ("Grabbing?"=w321:bool)
        n96 = case shown="False" w321 {
          tunnel: [w328 w340] -> w323
          tunnel: w322 -> [w328 w339]
          tunnel: w320 -> [_ w334]
          tunnel: w319 -> [w327 w333]
          tunnel: [w327 w332] -> w318
          tunnel: [w326 w329] -> w317
          frame False {
            w326 = T9[] [] items=["[Data] Default", "[Data] Update Graph", "[Pane] Calculate Size from Coord Change", "[Pane] Calculate Size from Display State", "[Plot] Redraw Frame", "[Plot] Update Plot Color", "[Scale] Autoscale or Crop X, Y, Z", "[Scale] Resize Scales", "[Scale] Align Scale Labels", "[Plot] Initialize Plot", "[Scale] X Scale", "[Scale] Y Scale", "[Scale] Z Scale", "[Scale] Multiplier/Offset", "[Scale] Name", "[Scale] Visible", "[Scale] Label Visible", "[Scale] Format"] ("Execution Tasks")
          }
          frame True {
            w329 = T9[] [enum."[Pane] Calculate Size from Coord Change", enum."[Scale] Resize Scales", enum."[Scale] Align Scale Labels", enum."[Plot] Redraw Frame", enum."[Data] Update Graph"] items=["[Data] Default", "[Data] Update Graph", "[Pane] Calculate Size from Coord Change", "[Pane] Calculate Size from Display State", "[Plot] Redraw Frame", "[Plot] Update Plot Color", "[Scale] Autoscale or Crop X, Y, Z", "[Scale] Resize Scales", "[Scale] Align Scale Labels", "[Plot] Initialize Plot", "[Scale] X Scale", "[Scale] Y Scale", "[Scale] Z Scale", "[Scale] Multiplier/Offset", "[Scale] Name", "[Scale] Visible", "[Scale] Label Visible", "[Scale] Format"] ("Execution Tasks")
            n97 = Unbundle By Name(w334) -> ("Refnum"=w337:refnum<vi>)
            n98 = property class="Ctl"(reference=w337) -> ("OwningVI"=w336:refnum<vi>)  [unwired: 1 in, 2 out]
            n99 = Bundle By Name(cluster=w339, "Grabbing?"=FALSE) -> (w340:T8)
            n100 = call-poly <vilib>:"Set Cursor.vi"("VI reference (current VI)"=w336, "icon"=u16 0) -> ()  [unwired: 8 in, 2 out]
            n101 = Bundle By Name(cluster=w333, "Action Name"="Perspective Change", "State Changed?"=TRUE) -> (w332:T5)
          }
        }
      }
      event "background": Mouse Down? {
        n102 = event-data() -> ()  [unwired: 1 in, 1 out]
        n103 = event-data() -> ()  [unwired: 2 in, 1 out]
        "background" <- FALSE ("background")
      }
      event "background": Mouse Up {
        # "attempt to save color if they apply paint brush without opening color palette"
        n104 = event-data() -> ()  [unwired: 1 in, 1 out]
        n105 = property on="background" class="Bool"() -> ("Colors [4]"=w348:cluster{u32, u32}[])  [unwired: 2 in, 2 out]
        n106 = Index Array(array=w348) -> (element=w347:cluster{u32, u32})  [unwired: 1 in]
        n107 = Unbundle(w347) -> (w346:u32)  [unwired: 1 out]
        n108 = Unbundle By Name(w354) -> ("Decor color"=w350:u32)
        n109 = Not Equal?(x=w350, y=w346) -> (x != y?=w349:bool)
        n110 = Bundle By Name(cluster=w352, "State Changed?"=w349) -> (w351:T5)
        n111 = Bundle By Name(cluster=w354, "Decor color"=w346) -> (w353:T6)
      }
      event "XY Scale Graph": Scale Range Change {
        w357 = T9[] [enum."[Scale] Autoscale or Crop X, Y, Z", enum."[Data] Update Graph"] items=["[Data] Default", "[Data] Update Graph", "[Pane] Calculate Size from Coord Change", "[Pane] Calculate Size from Display State", "[Plot] Redraw Frame", "[Plot] Update Plot Color", "[Scale] Autoscale or Crop X, Y, Z", "[Scale] Resize Scales", "[Scale] Align Scale Labels", "[Plot] Initialize Plot", "[Scale] X Scale", "[Scale] Y Scale", "[Scale] Z Scale", "[Scale] Multiplier/Offset", "[Scale] Name", "[Scale] Visible", "[Scale] Label Visible", "[Scale] Format"] ("Execution Tasks")
        n112 = event-data() -> ("NewRange.Maximum"=w370:dbl, "NewRange.Minimum"=w369:dbl, "Kind"=w375:enum16{"X-Scale", "Y-Scale", "Z-Scale"})  [unwired: 1 in]
        n113 = Unbundle By Name(w358) -> ("out of state queue"=w362:refnum<queue>)
        n114 = Dequeue Element(queue=w362) -> (queue out=w360:refnum<queue>, element=w361:T10)  [unwired: 2 in, 2 out]
        n115 = case shown="\"X-Scale\", Default" w375 {
          tunnel: w358 -> [w388 w402]
          tunnel: [w386 w400] -> w359
          tunnel: w370 -> [w382 w397]
          tunnel: w369 -> [w381 w396]
          tunnel: [w379 w394] -> w366
          tunnel: [w380 w393] -> w365
          tunnel: [enum16{"X-Scale", "Y-Scale", "Z-Scale"}."X-Scale" ("Kind") enum16{"X-Scale", "Y-Scale", "Z-Scale"}."Y-Scale" ("Kind")] -> w363
          tunnel: w361 -> [w387 w401]
          frame "X-Scale", Default {
            n116 = Unbundle By Name(w388) -> ("X-Axis Scaling Factor.Multiplier"=w384:dbl, "X-Axis Scaling Factor.Offset"=w383:dbl)
            n117 = call <vilib>:"svx_XYZ Scale.vi"("Minimum"=w381, "Maximum"=w382, "Offset"=w383, "Multiplier"=w384) -> ("Scaled.Minimum"=w379:dbl, "Scaled.Maximum"=w380:dbl, "Range.Minimum"=w378:dbl, "Range.Maximum"=w377:dbl, "flipped?"=w385:bool)  [unwired: 3 in]
            n118 = property on="XY Scale Graph" class="WFGraph (strict)"("XScale.Flipped"=w385) -> ()  [unwired: 2 in, 2 out]
            n119 = Bundle By Name(cluster=w387, "AutoScale X"=u8 0, "X-Axis Range.Maximum"=w377, "X-Axis Range.Minimum"=w378, "X-Axis Range Scaled.Minimum"=w379, "X-Axis Range Scaled.Maximum"=w380) -> (w386:T10)
          }
          frame "Y-Scale" {
            n120 = Unbundle By Name(w402) -> ("Y-Axis Scaling Factor.Multiplier"=w399:dbl, "Y-Axis Scaling Factor.Offset"=w398:dbl)
            n121 = call <vilib>:"svx_XYZ Scale.vi"("Minimum"=w396, "Maximum"=w397, "Offset"=w398, "Multiplier"=w399) -> ("Scaled.Minimum"=w394:dbl, "Scaled.Maximum"=w393:dbl, "Range.Minimum"=w392:dbl, "Range.Maximum"=w391:dbl, "flipped?"=w395:bool)  [unwired: 3 in]
            n122 = property on="XY Scale Graph" class="WFGraph (strict)"("YScale.Flipped"=w395) -> ()  [unwired: 2 in, 2 out]
            n123 = Bundle By Name(cluster=w401, "AutoScale Y"=u8 0, "Y-Axis Range.Maximum"=w391, "Y-Axis Range.Minimum"=w392, "Y-Axis Range Scaled.Minimum"=w394, "Y-Axis Range Scaled.Maximum"=w393) -> (w400:T10)
          }
        }
        n124 = Bundle By Name(cluster=w374, "Action Name"="Range Change", "State Changed?"=TRUE) -> (w373:T5)
        n125 = Unbundle By Name(w358) -> ("Scale Range Change"=w367:refnum<user-event>)
        n126 = Bundle("Scaled.Minimum"=w366, "Scaled.Maximum"=w365, "Kind"=w363) -> (w364:T11)  [unwired: 1 in]
        n127 = Enqueue Element(queue=w360, element=w359) -> ()  [unwired: 2 in, 3 out]
        n128 = Generate User Event(user event=w367, event data cluster=w364) -> ()  [unwired: 2 in, 2 out]
      }
      event "Z Scale Graph": Scale Range Change {
        w414 = T9[] [enum."[Scale] Autoscale or Crop X, Y, Z", enum."[Data] Update Graph"] items=["[Data] Default", "[Data] Update Graph", "[Pane] Calculate Size from Coord Change", "[Pane] Calculate Size from Display State", "[Plot] Redraw Frame", "[Plot] Update Plot Color", "[Scale] Autoscale or Crop X, Y, Z", "[Scale] Resize Scales", "[Scale] Align Scale Labels", "[Plot] Initialize Plot", "[Scale] X Scale", "[Scale] Y Scale", "[Scale] Z Scale", "[Scale] Multiplier/Offset", "[Scale] Name", "[Scale] Visible", "[Scale] Label Visible", "[Scale] Format"] ("Execution Tasks")
        # "Make sure scale is never flipped"
        # "If user flips scale from how the scale should be,\nflip the data."
        n129 = event-data() -> ("NewRange.Maximum"=w409:dbl, "NewRange.Minimum"=w408:dbl)  [unwired: 1 in]
        n130 = Unbundle By Name(w415) -> ("Z-Axis Scaling Factor.Multiplier"=w411:dbl, "Z-Axis Scaling Factor.Offset"=w410:dbl)
        n131 = Unbundle By Name(w415) -> ("out of state queue"=w419:refnum<queue>)
        n132 = Unbundle By Name(w415) -> ("Scale Range Change"=w422:refnum<user-event>)
        n133 = Dequeue Element(queue=w419) -> (queue out=w416:refnum<queue>, element=w418:T10)  [unwired: 2 in, 2 out]
        n134 = call <vilib>:"svx_XYZ Scale.vi"("Minimum"=w408, "Maximum"=w409, "Offset"=w410, "Multiplier"=w411) -> ("Scaled.Minimum"=w406:dbl, "Scaled.Maximum"=w405:dbl, "Range.Minimum"=w413:dbl, "Range.Maximum"=w412:dbl, "flipped?"=w407:bool)  [unwired: 3 in]
        n135 = property on="Z Scale Graph" class="WFGraph (strict)"("YScale.Flipped"=w407) -> ()  [unwired: 2 in, 2 out]
        n136 = Bundle By Name(cluster=w418, "AutoScale Z"=u8 0, "Z-Axis Range.Maximum"=w412, "Z-Axis Range.Minimum"=w413, "Z-Axis Range Scaled.Maximum"=w405, "Z-Axis Range Scaled.Minimum"=w406) -> (w417:T10)
        n137 = Bundle("Range.Minimum"=w413, "Range.Maximum"=w412, "Kind"=enum16{"X-Scale", "Y-Scale", "Z-Scale"}."Z-Scale") -> (w421:T12)  [unwired: 1 in]
        n138 = Generate User Event(user event=w422, event data cluster=w421) -> ()  [unwired: 2 in, 2 out]
        n139 = Bundle By Name(cluster=w427, "Action Name"="Range Change", "State Changed?"=TRUE) -> (w426:T5)
        n140 = Enqueue Element(queue=w416, element=w417) -> ()  [unwired: 2 in, 3 out]
      }
      event Pane Size {
        w430 = T9[] [enum."[Pane] Calculate Size from Display State", enum."[Scale] Resize Scales", enum."[Scale] Align Scale Labels", enum."[Plot] Redraw Frame", enum."[Data] Update Graph"] items=["[Data] Default", "[Data] Update Graph", "[Pane] Calculate Size from Coord Change", "[Pane] Calculate Size from Display State", "[Plot] Redraw Frame", "[Plot] Update Plot Color", "[Scale] Autoscale or Crop X, Y, Z", "[Scale] Resize Scales", "[Scale] Align Scale Labels", "[Plot] Initialize Plot", "[Scale] X Scale", "[Scale] Y Scale", "[Scale] Z Scale", "[Scale] Multiplier/Offset", "[Scale] Name", "[Scale] Visible", "[Scale] Label Visible", "[Scale] Format"] ("Execution Tasks")
        n141 = event-data() -> ("NewBnds"=w434:T13)  [unwired: 1 in]
        n142 = stacked-sequence {
          tunnel: w434 -> [_ w447 _]
          frame #0 {
            n143 = control-ref of="This VI"() -> (w436:refnum<vi>)
            n144 = property class="FcdVI"(reference=w436) -> (error out=w437:errorcluster, "Panel"=w439:refnum<vi>)  [unwired: 1 in, 1 out]
            n145 = property class="Pnl"(reference=w439, error in=w437, "DeferPanUpdts"=TRUE ("Defer Panel Updates")) -> ()  [unwired: 2 out]
          }
          frame #1 {
            # "-1 because 3D box was being cutoff by one pixel at the bottom"
            n146 = Unbundle By Name(w447) -> ("Right"=w446:i16, "Left"=w445:i16, "Bottom"=w444:i16, "Top"=w443:i16)
            n147 = Subtract(x=w446, y=w445) -> (x-y=w441:i16)
            n148 = Subtract(x=w444, y=w443) -> (x-y=w442:i16)
            n149 = Subtract(x=w441, y=i16 150 ("Width Offset")) -> (x-y=w449:i16)
            n150 = Subtract(x=w442, y=i16 60 ("Height Offset")) -> (x-y=w448:i16)
            n151 = property on="XY Graph" class="XYGraph (strict)"("Width"=w449, "Height"=w448) -> ()  [unwired: 2 in, 2 out]
            n152 = Decrement(x=w442) -> (x-1=w440:i16)
            n153 = property on="background" class="Bool"("Width"=w441, "Height"=w440) -> ()  [unwired: 2 in, 2 out]
          }
          frame #2 {
            # "Reposition Scales"
            n154 = property on="XY Scale Graph" class="WFGraph (strict)"() -> ("Plot Bounds"=w470:T13, "Position"=w464:T14)  [unwired: 2 in, 2 out]
            n155 = property on="XY Graph" class="XYGraph (strict)"() -> ("Plot Bounds"=w471:T13)  [unwired: 2 in, 2 out]
            n156 = property on="Z Scale Graph" class="WFGraph (strict)"() -> ("Position"=w454:T14, "Plot Bounds"=w459:T13)  [unwired: 2 in, 2 out]
            n157 = Unbundle By Name(w471) -> ("Right"=w461:i16, "Left"=w462:i16, "Bottom"=w460:i16)
            n158 = Unbundle By Name(w470) -> ("Left"=w469:i16, "Bottom"=w468:i16)
            n159 = Unbundle By Name(w459) -> ("Right"=w458:i16, "Bottom"=w457:i16)
            n160 = Bundle("Right"=w458, "Bottom"=w457) -> (w456:cluster{"Right":i16, "Bottom":i16})  [unwired: 1 in]
            n161 = Bundle("Right"=w461, "Bottom"=w460) -> (w455:cluster{"Right":i16, "Bottom":i16})  [unwired: 1 in]
            n162 = Bundle("Left"=w462, "Bottom"=w460) -> (w467:cluster{"Left":i16, "Bottom":i16})  [unwired: 1 in]
            n163 = Bundle("Left"=w469, "Bottom"=w468) -> (w466:cluster{"Left":i16, "Bottom":i16})  [unwired: 1 in]
            n164 = Subtract(x=w456, y=w455) -> (x-y=w453:cluster{"Right":i16, "Bottom":i16})
            n165 = Subtract(x=w467, y=w466) -> (x-y=w465:cluster{"Left":i16, "Bottom":i16})
            n166 = Subtract(x=w454, y=w453) -> (x-y=w452:T14)
            n167 = Add(x=w465, y=w464) -> (x+y=w463:T14)
            n168 = property on="Z Scale Graph" class="WFGraph (strict)"("Position"=w452) -> ()  [unwired: 2 in, 2 out]
            n169 = property on="XY Scale Graph" class="WFGraph (strict)"("Position"=w463) -> ()  [unwired: 2 in, 2 out]
          }
        }
      }
      event "Z Scale Graph", "XY Graph", "XY Scale Graph": Shortcut Menu Activation? {
        n170 = event-data() -> ("Coords"=→"Coords":T1, "CtlRef"=w477:refnum<vi>, "MenuRef"=w476:refnum<k9>)  [unwired: 1 in]
        n171 = control-ref of="XY Graph"() -> (w478:refnum<vi>)
        n172 = Not Equal?(x=w478, y=w477) -> (x != y?=w475:bool)
        n173 = call <vilib>:"svx_Shortcut Menu.vi"("waveform graph?"=w475, "Container State"=w473, "Display State In"=w474, "menu reference in"=w476) -> ()  [unwired: 7 in, 1 out]
        n174 = event-data() -> ()  [unwired: 2 in, 1 out]
      }
      event Shortcut Menu Activation? {
        # "Delete unwanted menu items"
        n175 = event-data() -> ("Coords"=w482:T1, "MenuRef"=w488:refnum<k9>)  [unwired: 1 in]
        n176 = local write "Coords"(w482) -> ()
        n177 = for {
          tunnel: cluster{"menu tag":string, string[]}[] [{"menu tag"="APP_SC_ADVANCED", ["APP_SC_KEY_NAVIGATION", "APP_SC_CUSTOMIZE", "APP_SC_SHOW_DIAGRAM"]}, {"menu tag"="", ["APP_SC_PROPERTIES", "APP_SC_SHOW_DIAGRAM"]}] -> [w498] mode=indexing
          shift-right: [w495] -> w484
          shift-left: w488 -> [w499]
          n178 = Unbundle(w498) -> ("menu tag"=w497:string, w496:string[])
          n179 = Delete Menu Items(7:w496, 8:w497, 9:w499) -> (3:w495:refnum<k9>)  [unwired: 1 in, 1 out]
        }
        n180 = Unbundle By Name(w483) -> ("Run Mode?"=w485:bool)
        n181 = case shown="False" w485 {
          tunnel: w484 -> [w492 _]
          frame False {
            n182 = Insert Menu Items(7:string[] ["SV_WF_PROPERTIES"], 8:string[] ["Properties"], 9:w492) -> ()  [unwired: 3 in, 3 out]
          }
          frame True {
          }
        }
        n183 = event-data() -> ()  [unwired: 2 in, 1 out]
      }
      event "Z Scale Graph", "XY Graph", "XY Scale Graph": Shortcut Menu Selection (User) {
        n184 = event-data() -> ("ItemTag"=w508:string)  [unwired: 1 in]
        n185 = case shown="\"SV_WF_PROPERTIES\"" w508 {
          tunnel: w506 -> [w509 w517 w527 w537 w542 w562 w580 w601 w612 w622 w637 w646]
          tunnel: [w509 w516 w526 w536 w542 w562 w580 w602 w613 w619 w637 w646] -> w505
          tunnel: [w510 w518 w528 w538 w557 w574 w593 w604 w615 w632 w641 w650] -> w503
          tunnel: w504 -> [w510 w519 w529 w539 w558 w575 w592 w603 w614 w631 w640 w649]
          tunnel: w502 -> [_ _ _ _ _ _ _ _ _ w630 _ _]
          tunnel: w501 -> [_ _ _ _ _ _ _ _ _ w629 w639 w648]
          tunnel: [_ _ _ _ w541 w559 w577 w595 w606 w618 _ _] -> w500
          frame Default {
          }
          frame "SV_WF_VISIBLE_ITEMS_X_SCALE" {
            n186 = Unbundle By Name(w517) -> ("X-Scale Visible"=w515:bool)
            n187 = Not(x=w515) -> (.not. x?=w512:bool)
            n188 = Bundle By Name(cluster=w517, "X-Scale Visible"=w512) -> (w516:T6)
            n189 = property on="XY Scale Graph" class="WFGraph (strict)"("XScale.Visible"=w512) -> ()  [unwired: 2 in, 2 out]
            n190 = Select(t="Show X Scale" ("Action Name"), s=w512, f="Hide X Scale") -> (s? t:f=w514:string)
            n191 = Bundle By Name(cluster=w519, "Action Name"=w514, "State Changed?"=TRUE) -> (w518:T5)
          }
          frame "SV_WF_VISIBLE_ITEMS_Y_SCALE" {
            n192 = Unbundle By Name(w527) -> ("Y-Scale Visible"=w525:bool)
            n193 = Not(x=w525) -> (.not. x?=w522:bool)
            n194 = Bundle By Name(cluster=w527, "Y-Scale Visible"=w522) -> (w526:T6)
            n195 = property on="XY Scale Graph" class="WFGraph (strict)"("YScale.Visible"=w522) -> ()  [unwired: 2 in, 2 out]
            n196 = Select(t="Show Y Scale" ("Action Name"), s=w522, f="Hide Y Scale") -> (s? t:f=w521:string)
            n197 = Bundle By Name(cluster=w529, "Action Name"=w521, "State Changed?"=TRUE) -> (w528:T5)
          }
          frame "SV_WF_VISIBLE_ITEMS_Z_SCALE" {
            n198 = Unbundle By Name(w537) -> ("Z-Scale Visible"=w535:bool)
            n199 = Not(x=w535) -> (.not. x?=w532:bool)
            n200 = Bundle By Name(cluster=w537, "Z-Scale Visible"=w532) -> (w536:T6)
            n201 = property on="Z Scale Graph" class="WFGraph (strict)"("YScale.Visible"=w532) -> ()  [unwired: 2 in, 2 out]
            n202 = Select(t="Show Z Scale" ("Action Name"), s=w532, f="Hide Z Scale") -> (s? t:f=w531:string)
            n203 = Bundle By Name(cluster=w539, "Action Name"=w531, "State Changed?"=TRUE) -> (w538:T5)
          }
          frame "SV_WF_AUTOSCALE_X" {
            w541 = T9[] [enum."[Scale] Autoscale or Crop X, Y, Z", enum."[Data] Update Graph"] items=["[Data] Default", "[Data] Update Graph", "[Pane] Calculate Size from Coord Change", "[Pane] Calculate Size from Display State", "[Plot] Redraw Frame", "[Plot] Update Plot Color", "[Scale] Autoscale or Crop X, Y, Z", "[Scale] Resize Scales", "[Scale] Align Scale Labels", "[Plot] Initialize Plot", "[Scale] X Scale", "[Scale] Y Scale", "[Scale] Z Scale", "[Scale] Multiplier/Offset", "[Scale] Name", "[Scale] Visible", "[Scale] Label Visible", "[Scale] Format"] ("Execution Tasks")
            n204 = Unbundle By Name(w542) -> ("out of state queue"=w546:refnum<queue>)
            n205 = Dequeue Element(queue=w546) -> (queue out=w545:refnum<queue>, element=w544:T10)  [unwired: 2 in, 2 out]
            n206 = Unbundle By Name(w544) -> ("AutoScale X"=w552:u8)
            n207 = Equal?(x=w552, y=u8 2) -> (x = y?=w548:bool)
            n208 = Select(t=u8 0 ("y"), s=w548, f=u8 2 ("y")) -> (s? t:f=w551:u8)
            n209 = Bundle By Name(cluster=w544, "AutoScale X"=w551) -> (w543:T10)
            n210 = Select(t="Autoscale Deselection" ("Action Name"), s=w548, f="Autoscale Selection") -> (s? t:f=w547:string)
            n211 = Bundle By Name(cluster=w558, "Action Name"=w547, "State Changed?"=TRUE) -> (w557:T5)
            n212 = Enqueue Element(queue=w545, element=w543) -> ()  [unwired: 2 in, 3 out]
          }
          frame "SV_WF_AUTOSCALE_Y" {
            w559 = T9[] [enum."[Scale] Autoscale or Crop X, Y, Z", enum."[Data] Update Graph"] items=["[Data] Default", "[Data] Update Graph", "[Pane] Calculate Size from Coord Change", "[Pane] Calculate Size from Display State", "[Plot] Redraw Frame", "[Plot] Update Plot Color", "[Scale] Autoscale or Crop X, Y, Z", "[Scale] Resize Scales", "[Scale] Align Scale Labels", "[Plot] Initialize Plot", "[Scale] X Scale", "[Scale] Y Scale", "[Scale] Z Scale", "[Scale] Multiplier/Offset", "[Scale] Name", "[Scale] Visible", "[Scale] Label Visible", "[Scale] Format"] ("Execution Tasks")
            n213 = Unbundle By Name(w562) -> ("out of state queue"=w564:refnum<queue>)
            n214 = Dequeue Element(queue=w564) -> (queue out=w563:refnum<queue>, element=w560:T10)  [unwired: 2 in, 2 out]
            n215 = Unbundle By Name(w560) -> ("AutoScale Y"=w573:u8)
            n216 = Equal?(x=w573, y=u8 2) -> (x = y?=w567:bool)
            n217 = Select(t=u8 0 ("y"), s=w567, f=u8 2 ("y")) -> (s? t:f=w569:u8)
            n218 = Select(t="Autoscale Deselection" ("Action Name"), s=w567, f="Autoscale Selection") -> (s? t:f=w565:string)
            n219 = Bundle By Name(cluster=w575, "Action Name"=w565, "State Changed?"=TRUE) -> (w574:T5)
            n220 = Bundle By Name(cluster=w560, "AutoScale Y"=w569) -> (w561:T10)
            n221 = Enqueue Element(queue=w563, element=w561) -> ()  [unwired: 2 in, 3 out]
          }
          frame "SV_WF_AUTOSCALE_Z" {
            w577 = T9[] [enum."[Scale] Autoscale or Crop X, Y, Z", enum."[Data] Update Graph"] items=["[Data] Default", "[Data] Update Graph", "[Pane] Calculate Size from Coord Change", "[Pane] Calculate Size from Display State", "[Plot] Redraw Frame", "[Plot] Update Plot Color", "[Scale] Autoscale or Crop X, Y, Z", "[Scale] Resize Scales", "[Scale] Align Scale Labels", "[Plot] Initialize Plot", "[Scale] X Scale", "[Scale] Y Scale", "[Scale] Z Scale", "[Scale] Multiplier/Offset", "[Scale] Name", "[Scale] Visible", "[Scale] Label Visible", "[Scale] Format"] ("Execution Tasks")
            n222 = Unbundle By Name(w580) -> ("out of state queue"=w582:refnum<queue>)
            n223 = Dequeue Element(queue=w582) -> (queue out=w581:refnum<queue>, element=w578:T10)  [unwired: 2 in, 2 out]
            n224 = Unbundle By Name(w578) -> ("AutoScale Z"=w588:u8)
            n225 = Equal?(x=w588, y=u8 2) -> (x = y?=w584:bool)
            n226 = Select(t=u8 0 ("y"), s=w584, f=u8 2 ("y")) -> (s? t:f=w587:u8)
            n227 = Select(t="Autoscale Deselection" ("Action Name"), s=w584, f="Autoscale Selection") -> (s? t:f=w583:string)
            n228 = Bundle By Name(cluster=w578, "AutoScale Z"=w587) -> (w579:T10)
            n229 = Bundle By Name(cluster=w592, "Action Name"=w583, "State Changed?"=TRUE) -> (w593:T5)
            n230 = Enqueue Element(queue=w581, element=w579) -> ()  [unwired: 2 in, 3 out]
          }
          frame "SV_WF_PLOT_TRANSPARENCY" {
            w595 = T9[] [enum."[Plot] Update Plot Color"] items=["[Data] Default", "[Data] Update Graph", "[Pane] Calculate Size from Coord Change", "[Pane] Calculate Size from Display State", "[Plot] Redraw Frame", "[Plot] Update Plot Color", "[Scale] Autoscale or Crop X, Y, Z", "[Scale] Resize Scales", "[Scale] Align Scale Labels", "[Plot] Initialize Plot", "[Scale] X Scale", "[Scale] Y Scale", "[Scale] Z Scale", "[Scale] Multiplier/Offset", "[Scale] Name", "[Scale] Visible", "[Scale] Label Visible", "[Scale] Format"] ("Execution Tasks")
            # "Reversed because we want\nto do the opposite of the previous selection"
            n231 = Unbundle By Name(w601) -> ("Plot Transparency"=w597:bool)
            n232 = Not(x=w597) -> (.not. x?=w596:bool)
            n233 = Select(t="Plot Transparency Deselection" ("Action Name"), s=w597, f="Plot Transparency Selection") -> (s? t:f=w598:string)
            n234 = Bundle By Name(cluster=w601, "Plot Transparency"=w596) -> (w602:T6)
            n235 = Bundle By Name(cluster=w603, "Action Name"=w598, "State Changed?"=TRUE) -> (w604:T5)
          }
          frame "SV_REVERSE_ORDER" {
            w606 = T9[] [enum."[Scale] Autoscale or Crop X, Y, Z", enum."[Data] Update Graph"] items=["[Data] Default", "[Data] Update Graph", "[Pane] Calculate Size from Coord Change", "[Pane] Calculate Size from Display State", "[Plot] Redraw Frame", "[Plot] Update Plot Color", "[Scale] Autoscale or Crop X, Y, Z", "[Scale] Resize Scales", "[Scale] Align Scale Labels", "[Plot] Initialize Plot", "[Scale] X Scale", "[Scale] Y Scale", "[Scale] Z Scale", "[Scale] Multiplier/Offset", "[Scale] Name", "[Scale] Visible", "[Scale] Label Visible", "[Scale] Format"] ("Execution Tasks")
            n236 = Unbundle By Name(w612) -> ("Rev Z Order"=w608:bool)
            n237 = Not(x=w608) -> (.not. x?=w611:bool)
            n238 = Select(t="Reverse Order Deselection" ("Action Name"), s=w608, f="Reverse Order Selection") -> (s? t:f=w607:string)
            n239 = Bundle By Name(cluster=w612, "Rev Z Order"=w611) -> (w613:T6)
            n240 = Bundle By Name(cluster=w614, "Action Name"=w607, "State Changed?"=TRUE) -> (w615:T5)
          }
          frame "SV_WF_PROPERTIES" {
            w618 = T9[] [enum."[Scale] Autoscale or Crop X, Y, Z", enum."[Data] Update Graph"] items=["[Data] Default", "[Data] Update Graph", "[Pane] Calculate Size from Coord Change", "[Pane] Calculate Size from Display State", "[Plot] Redraw Frame", "[Plot] Update Plot Color", "[Scale] Autoscale or Crop X, Y, Z", "[Scale] Resize Scales", "[Scale] Align Scale Labels", "[Plot] Initialize Plot", "[Scale] X Scale", "[Scale] Y Scale", "[Scale] Z Scale", "[Scale] Multiplier/Offset", "[Scale] Name", "[Scale] Visible", "[Scale] Label Visible", "[Scale] Format"] ("Execution Tasks")
            n241 = call <vilib>:"svx_Waterfall QueueToState.vi"("State In"=w622) -> ("State Out"=w621:T6)  [unwired: 10 in]
            n242 = control-ref of="XY Scale Graph"() -> (w627:refnum<vi>)
            n243 = control-ref of="Z Scale Graph"() -> (w626:refnum<vi>)
            n244 = control-ref of="XY Graph"() -> (w617:refnum<vi>)
            n245 = Unbundle By Name(w629) -> ("Refnum"=w628:refnum<vi>)
            n246 = call <vilib>:"svx_Property Page.vi"("Z Scale Graph Refnum"=w626, "XY Graph Reference"=w617, "XY Scale Graph Refnum"=w627, "Container Refnum"=w628, "State in"=w621, "Data In"=w630) -> ("Cancel?"=w624:bool, "State out"=w620:T6)  [unwired: 4 in]
            n247 = Not(x=w624) -> (.not. x?=w625:bool)
            n248 = Bundle By Name(cluster=w631, "Action Name"="Property Page Changes", "State Changed?"=w625) -> (w632:T5)
            n249 = call <vilib>:"svx_Waterfall StateToQueue.vi"("Display State In"=w620) -> ("Display State Out"=w619:T6)  [unwired: 10 in]
          }
          frame "APP_SC_LABEL" {
            n250 = Unbundle By Name(w639) -> ("Refnum"=w636:refnum<vi>)
            n251 = property class="Ctl"(reference=w636) -> (reference out=w633:refnum<vi>, "Label.Visible"=w635:bool)  [unwired: 1 in, 1 out]
            n252 = Not(x=w635) -> (.not. x?=w634:bool)
            n253 = property class="Ctl"(reference=w633, "Label.Visible"=w634) -> ()  [unwired: 1 in, 2 out]
            n254 = Bundle By Name(cluster=w640, "Action Name"="Label Visability") -> (w641:T5)
          }
          frame "APP_SC_CAPTION" {
            n255 = Unbundle By Name(w648) -> ("Refnum"=w645:refnum<vi>)
            n256 = property class="Ctl"(reference=w645) -> (reference out=w642:refnum<vi>, "Caption.Visible"=w644:bool)  [unwired: 1 in, 1 out]
            n257 = Not(x=w644) -> (.not. x?=w643:bool)
            n258 = property class="Ctl"(reference=w642, "Caption.Visible"=w643) -> ()  [unwired: 1 in, 2 out]
            n259 = Bundle By Name(cluster=w649, "Action Name"="Caption Visability") -> (w650:T5)
          }
        }
      }
      event "XY Scale Graph", "Z Scale Graph", "XY Graph": Shortcut Menu Selection? (App) {
        n260 = event-data() -> ("ItemTag"=w657:string)  [unwired: 1 in]
        n261 = case shown="\"APP_SC_CLEAR_GRAPH\"" w657 {
          tunnel: [FALSE ("Discard?") TRUE ("Discard?")] -> w656
          tunnel: w655 -> [w662 _]
          tunnel: [w662 T3 {"z0"=0.0, "dz"=1.0, "Plots"=[]} ("Data In")] -> w654
          tunnel: w653 -> [w661 w668]
          tunnel: [w661 w667] -> w652
          tunnel: [w660 w664] -> w651
          frame Default {
            w660 = T9[] [] items=["[Data] Default", "[Data] Update Graph", "[Pane] Calculate Size from Coord Change", "[Pane] Calculate Size from Display State", "[Plot] Redraw Frame", "[Plot] Update Plot Color", "[Scale] Autoscale or Crop X, Y, Z", "[Scale] Resize Scales", "[Scale] Align Scale Labels", "[Plot] Initialize Plot", "[Scale] X Scale", "[Scale] Y Scale", "[Scale] Z Scale", "[Scale] Multiplier/Offset", "[Scale] Name", "[Scale] Visible", "[Scale] Label Visible", "[Scale] Format"] ("Execution Tasks")
          }
          frame "APP_SC_CLEAR_GRAPH" {
            w664 = T9[] [enum."[Scale] Autoscale or Crop X, Y, Z", enum."[Data] Update Graph"] items=["[Data] Default", "[Data] Update Graph", "[Pane] Calculate Size from Coord Change", "[Pane] Calculate Size from Display State", "[Plot] Redraw Frame", "[Plot] Update Plot Color", "[Scale] Autoscale or Crop X, Y, Z", "[Scale] Resize Scales", "[Scale] Align Scale Labels", "[Plot] Initialize Plot", "[Scale] X Scale", "[Scale] Y Scale", "[Scale] Z Scale", "[Scale] Multiplier/Offset", "[Scale] Name", "[Scale] Visible", "[Scale] Label Visible", "[Scale] Format"] ("Execution Tasks")
            n262 = Bundle By Name(cluster=w668, "Action Name"="Clear Graph", "Data Changed?"=TRUE) -> (w667:T5)
          }
        }
        n263 = event-data("Discard?"=w656) -> ()  [unwired: 1 in, 1 out]
      }
      event Mouse Down? {
        n264 = event-data() -> ("Button"=w672:u16, "Mods"=w676:cluster{"Double Click":bool, "Menu Key":bool}, "PlatMods"=w674:T15, "Coords"=w671:T1)  [unwired: 1 in]
        n265 = case shown="1" w672 {
          tunnel: w676 -> [w685 w689]
          tunnel: [w688 w689] -> w675
          tunnel: w671 -> [w687 _]
          frame 1 {
            n266 = local read "Coords"() -> (w686:T1)
            n267 = Unbundle By Name(w685) -> ("Double Click"=w682:bool)
            n268 = Equal?(x=w687, y=w686) -> (x = y?=w683:bool)
            n269 = Select(t=FALSE ("Double Click"), s=w683, f=w682) -> (s? t:f=w681:bool)
            n270 = Bundle By Name(cluster=w685, "Double Click"=w681) -> (w688:cluster{"Double Click":bool, "Menu Key":bool})
          }
          frame 0, Default {
          }
        }
        n271 = event-data("Button"=w672, "Mods"=w675, "PlatMods"=w674, "Discard?"=FALSE) -> ()  [unwired: 1 in, 1 out]
      }
    }
    n272 = local read "Dec/Cropped and Lines"() -> (w15:T2)
    n273 = control-ref of="XY Scale Graph"() -> (w14:refnum<vi>)
    n274 = control-ref of="Z Scale Graph"() -> (w13:refnum<vi>)
    n275 = control-ref of="XY Graph"() -> (w8:refnum<vi>)
    n276 = control-ref of="background"() -> (w11:refnum<vi>)
    n277 = control-ref of="This VI"() -> (w12:refnum<vi>)
    n278 = call <vilib>:"svx_Waterfall Execute.vi"("Data In"=w20, "Display State In"=w23, "Container State"=w21, "Dec/Cropped and Lines"=w15, "Execution Tasks"=w17, "XY Graph Ref"=w8, "Coords"=w22, "XY Scale Graph ref"=w14, "Z Scale Graph ref"=w13, "This VI"=w12, "Background ref"=w11) -> ("Data Out"=w10:T3, "Display State Out"=w18:T6, "Dec/Cropped out"=→"Dec/Cropped and Lines":T2)  [unwired: 6 in]
  }
  "Display State Out" <- w4
  "Data Out" <- w7
  "Action" <- w2
  n279 = disable-structure shown="Enabled" {
    frame Disabled {
      # "Temporarily enable and run VI to reposition graphs"
      n280 = stacked-sequence {
        frame #0 {
          n281 = control-ref of="This VI"() -> (w690:refnum<vi>)
          n282 = property on="Pane" class="Pane"() -> ("Width"=w692:u32, "Height"=w691:u32)  [unwired: 2 in, 2 out]
          n283 = property on="Property Node" class="FcdVI"(reference=w690) -> ("Panel"=w699:refnum<vi>)  [unwired: 1 in, 2 out]
          n284 = Subtract(x=w692, y=i16 150 ("Width Offset")) -> (x-y=w695:u32)
          n285 = Subtract(x=w691, y=i16 60 ("Height Offset")) -> (x-y=w696:u32)
          n286 = property on="XY Graph" class="XYGraph (strict)"("Width"=w695, "Height"=w696) -> ()  [unwired: 2 in, 2 out]
          n287 = property on="Property Node" class="Pnl"(reference=w699) -> ("Decos[]"=w698:refnum<vi>[])  [unwired: 1 in, 2 out]
          n288 = Decrement(x=w691) -> (x-1=w700:u32)
          n289 = Index Array(array=w698) -> (element=w697:refnum<vi>)  [unwired: 1 in]
          n290 = property on="Property Node" class="Decor"(reference=w697, "Width"=w692, "Height"=w700) -> ()  [unwired: 1 in, 2 out]
        }
        frame #1 {
          n291 = property on="XY Scale Graph" class="WFGraph (strict)"() -> ("Plot Bounds"=w702:T13, "Position"=w708:T14)  [unwired: 2 in, 2 out]
          n292 = property on="XY Graph" class="XYGraph (strict)"() -> ("Plot Bounds"=w701:T13)  [unwired: 2 in, 2 out]
          n293 = property on="Z Scale Graph" class="WFGraph (strict)"() -> ("Position"=w718:T14, "Plot Bounds"=w713:T13)  [unwired: 2 in, 2 out]
          n294 = Unbundle By Name(w701) -> ("Right"=w711:i16, "Left"=w710:i16, "Bottom"=w712:i16)
          n295 = Unbundle By Name(w702) -> ("Left"=w703:i16, "Bottom"=w704:i16)
          n296 = Unbundle By Name(w713) -> ("Right"=w714:i16, "Bottom"=w715:i16)
          n297 = Bundle("Right"=w714, "Bottom"=w715) -> (w716:cluster{"Right":i16, "Bottom":i16})  [unwired: 1 in]
          n298 = Bundle("Right"=w711, "Bottom"=w712) -> (w717:cluster{"Right":i16, "Bottom":i16})  [unwired: 1 in]
          n299 = Bundle("Left"=w710, "Bottom"=w712) -> (w705:cluster{"Left":i16, "Bottom":i16})  [unwired: 1 in]
          n300 = Bundle("Left"=w703, "Bottom"=w704) -> (w706:cluster{"Left":i16, "Bottom":i16})  [unwired: 1 in]
          n301 = Subtract(x=w716, y=w717) -> (x-y=w719:cluster{"Right":i16, "Bottom":i16})
          n302 = Subtract(x=w705, y=w706) -> (x-y=w707:cluster{"Left":i16, "Bottom":i16})
          n303 = Subtract(x=w718, y=w719) -> (x-y=w720:T14)
          n304 = Add(x=w707, y=w708) -> (x+y=w709:T14)
          n305 = property on="Z Scale Graph" class="WFGraph (strict)"("Position"=w720) -> ()  [unwired: 2 in, 2 out]
          n306 = property on="XY Scale Graph" class="WFGraph (strict)"("Position"=w709) -> ()  [unwired: 2 in, 2 out]
        }
      }
    }
    frame Enabled {
      # "Enable this empty diagram"
    }
  }
  n307 = disable-structure shown="Enabled" {
    frame Disabled {
      # "Align Scale labels"
      n308 = property on="XY Scale Graph" class="WFGraph (strict)"() -> ("YScale.Top"=w732:i32, "YScale.Height"=w729:u32, "YScale.NameLbl.Height"=w730:u32)  [unwired: 2 in, 2 out]
      n309 = property on="XY Scale Graph" class="WFGraph (strict)"() -> ("XScale.Left"=w723:i32, "XScale.Width"=w724:u32, "XScale.NameLbl.Width"=w722:u32)  [unwired: 2 in, 2 out]
      n310 = Subtract(x=w729, y=w730) -> (x-y=w731:u32)
      n311 = Subtract(x=w724, y=w722) -> (x-y=w726:u32)
      n312 = Divide(x=w731, y=u32 2) -> (x/y=w733:dbl)
      n313 = Divide(x=w726, y=u32 2) -> (x/y=w725:dbl)
      n314 = Add(x=w732, y=w733) -> (x+y=w734:dbl)
      n315 = Add(x=w723, y=w725) -> (x+y=w721:dbl)
      n316 = property on="XY Scale Graph" class="WFGraph (strict)"("YScale.NameLbl.Top"=w734, "XScale.NameLbl.Left"=w721) -> ()  [unwired: 2 in, 2 out]
    }
    frame Enabled {
    }
  }
